vi "WPI_SimpleGyro_Get Rate.vi"(8 "error in":errorcluster, 11 "SimpleGyroDevRef":T1) -> (0 "error out":errorcluster, 1 "Calibrated?":bool, 2 "Rate":dbl, 3 "SimpleGyroDevRef":T1)   [LabVIEW 2014, in "SimpleGyro.lvlib"]
uses:
  SimpleGyro.lvlib
  WPI_SimpleGyroDevRef.ctl
  <vilib>/Rock Robotics/SystemInterfaces/Typedef/FPGA_TypedefDigitalModule.ctl
  <vilib>/Rock Robotics/SystemInterfaces/spilib/spi_bus.ctl
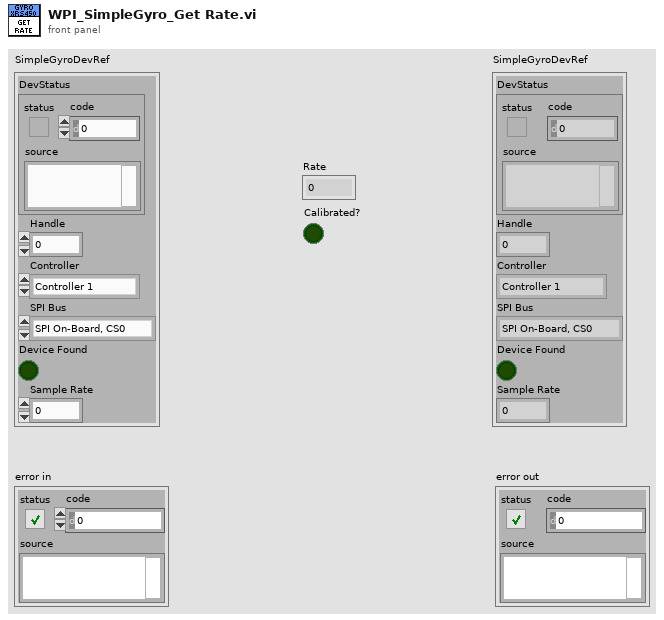
[diagram p1: front panel]
types:
  T1 = typedef "SimpleGyro.lvlib/WPI_SimpleGyroDevRef.ctl" = cluster{"DevStatus":errorcluster, "Handle":i32, "Controller":T2, "SPI Bus":T3, "Device Found":bool, "Sample Rate":dbl}
  T2 = typedef "FPGA_TypedefDigitalModule.ctl" = enum16{"Controller 1"}
  T3 = typedef "spi_bus.ctl" = enum16{"SPI On-Board, CS0", "SPI On-Board, CS1", "SPI On-Board, CS2", "SPI On-Board, CS3", "SPI MXP", "Invalid"}
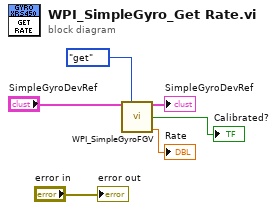
[diagram p0: block diagram]
diagram:
  n1 = call "WPI_SimpleGyroFGV.vi"("SimpleGyroDevRef"="SimpleGyroDevRef", "Operation"=enum16{"set", "get"}."get") -> ("SimpleGyroDevRef"=→"SimpleGyroDevRef":T1, "Calibrated?"=→"Calibrated?":bool, "Rate"=→"Rate":dbl)  [unwired: 9 in, 2 out]
  "error out" <- "error in"
